vi "Apply Application Style.vi"(8 "error in (no error)":errorcluster, 10 "VI Refnum":refnum<vi>, 11 "ApplicationStyleReference in":T1) -> (0 "error out":errorcluster)   [LabVIEW 2017, in "IViewable.lvlib" / "ApplicationStyleReference.lvclass"]
uses:
  ApplicationStyleReference.lvclass
  Application Style Reference.ctl
  ApplicationStyleReference.lvclass/ApplicationStyleReference.ctl
  IApplicationStyle/IApplicationStyle.lvclass
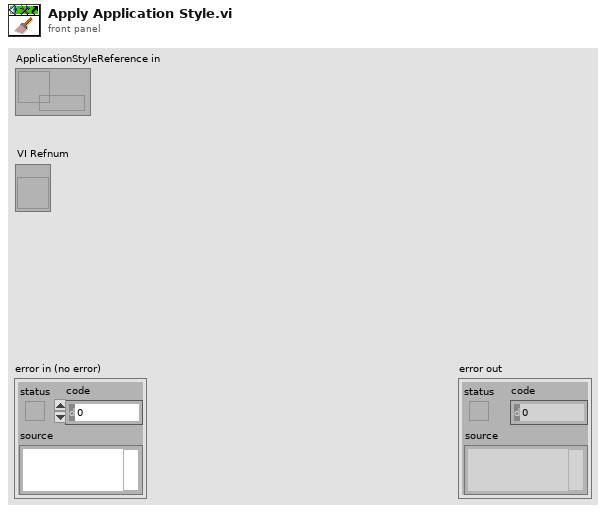
[diagram p1: front panel]
types:
  T1 = typedef "IViewable.lvlib/ApplicationStyleReference.lvclass/Application Style Reference.ctl" = refnum<data-value>
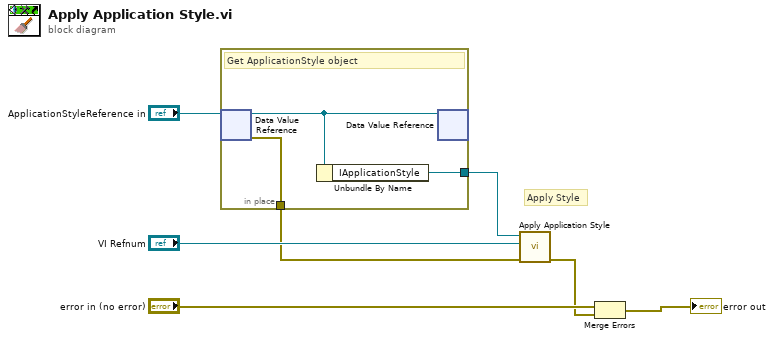
[diagram p0: block diagram]
diagram:
  # "Apply Style"
  n1 = in-place {
    in-place-border: [w9] -> w3
    in-place-border: [w8] -> w1
    # "Get ApplicationStyle object"
    n2 = in-place-dvr #1("ApplicationStyleReference in") -> (w10:refnum<class "ApplicationStyleReference.lvclass">, w8:errorcluster)
    n3 = Unbundle By Name(w10) -> ("IApplicationStyle"=w9:refnum<class "IApplicationStyle.lvclass">)
    n4 = in-place-dvr #1(w10) -> ()  [unwired: 2 out]
  }
  n5 = call-dynamic "Apply Application Style.vi"("error in (no error)"=w1, "VI Refnum"="VI Refnum", "IApplicationStyle in"=w3) -> ("error out"=w2:errorcluster)  [unwired: 8 in]
  n6 = Merge Errors("error in (no error)", w2) -> (→"error out":errorcluster)
